vi "test_has_position.vi"() -> ()   [LabVIEW 2022 SP3]
uses:
  <instrlib>/yaq/yaq_labview_error_handler.vi
  <vilib>/Utility/error.llb/Simple Error Handler.vi
panel:
  out "Current Position":dbl
  out "Destination":dbl
  in  "Set Relative":dbl
  in  "Set Position":dbl
  in  "stop":bool
  out "units":string
  out "busy?":bool
  in  "Python path":path=path "C:/ProgramData/Anaconda3/envs/lv4/pythonw.exe"
  in  "Python version":string="3.8.0"
  in  "Python Module Path":path=path "C:/Users/kamey/work/labview/yaq-labview/python/yaqc_labview.py"
  in  "Port":i32=39004
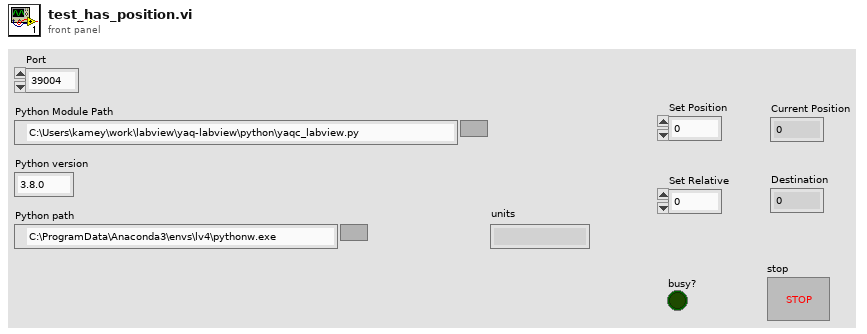
[diagram p1: front panel]
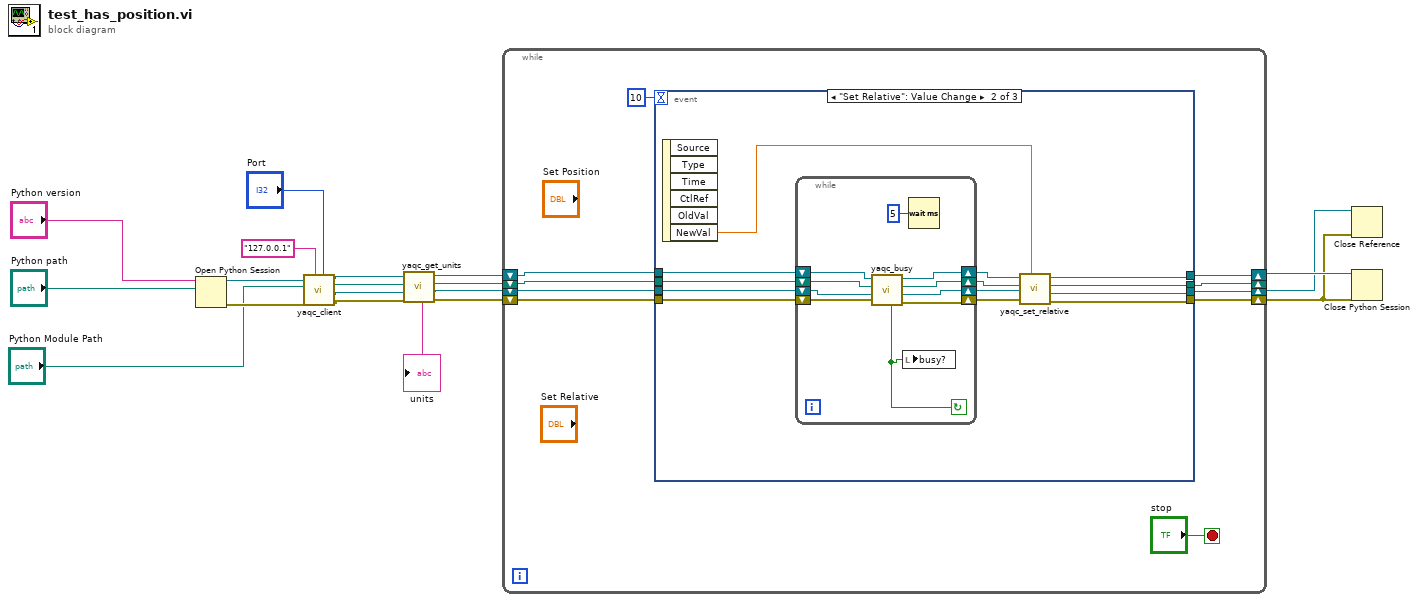
[diagram p0: block diagram]
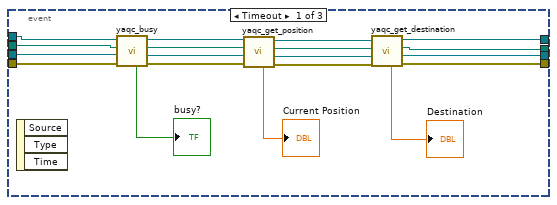
[diagram p2: hidden frame]
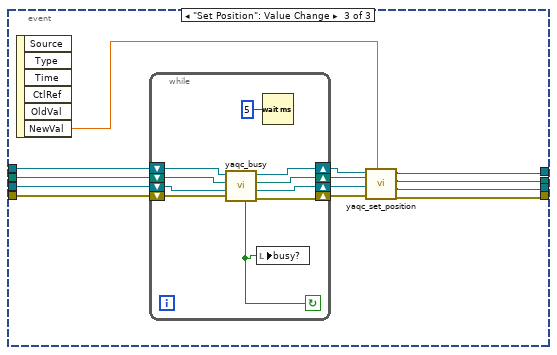
[diagram p3: hidden frame]
diagram:
  n1 = Open Python Session(python version="Python version", python path="Python path") -> (session out=w18:refnum<k35>, error out=w19:errorcluster)  [unwired: 1 in]
  n2 = call "yaqc_client.vi"("Port"="Port", "host ('127.0.0.1')"="127.0.0.1", "error in (no error)"=w19, "Python Module Path"="Python Module Path", "Python Session In"=w18) -> ("error out"=w4:errorcluster, "Yaqc Client"=w3:refnum<k38>, "Python Module Path Out"=w2:path, "Python Session Out"=w1:refnum<k35>)  [unwired: 3 in]
  n3 = call "yaqc_get_units.vi"("error in (no error)"=w4, "Yaqc Client In"=w3, "Python Module Path In"=w2, "Python Session In"=w1) -> ("error out"=w11:errorcluster, "Yaqc Client Out"=w10:refnum<k38>, "Python Module Path Out"=w9:path, "Python Session Out"=w8:refnum<k35>, "units"=→"units":string)  [unwired: 3 in]
  n4 = while {
    shift-right: [w26] -> w6
    shift-left: w11 -> [w28]
    shift-right: [w21] -> w5
    shift-left: w10 -> [w27]
    shift-right: [w22] -> _
    shift-left: w9 -> [w25]
    shift-right: [w23] -> w7
    shift-left: w8 -> [w24]
    stop <- "stop" stop-if-true
    n5 = event shown="[1] \"Set Relative\": Value Change" {
      selector: _ -> [_ _ _]
      dyn-events: _ -> [_ _ _]
      timeout: 10 -> [_ _ _]
      tunnel: w28 -> [w47 w61 w84]
      tunnel: w27 -> [w48 w60 w83]
      tunnel: [w44 w53 w80] -> w26
      tunnel: w25 -> [w43 w59 w82]
      tunnel: w24 -> [w42 w58 w81]
      tunnel: [w35 w50 w73] -> w23
      tunnel: [w34 w51 w75] -> w22
      tunnel: [w33 w52 w77] -> w21
      event Timeout {
        n6 = event-data() -> ()  [unwired: 1 in, 3 out]
        n7 = call "yaqc_busy.vi"("error in (no error)"=w47, "Yaqc Client In"=w48, "Python Module Path In"=w43, "Python Session In"=w42) -> ("error out"=w46:errorcluster, "Yaqc Client Out"=w38:refnum<k38>, "Python Module Path Out"=w39:path, "Python Session Out"=w41:refnum<k35>, "busy?"=→"busy?":bool)  [unwired: 3 in]
        n8 = call "yaqc_get_position.vi"("error in (no error)"=w46, "Yaqc Client In"=w38, "Python Module Path In"=w39, "Python Session In"=w41) -> ("error out"=w45:errorcluster, "Yaqc Client Out"=w37:refnum<k38>, "Python Module Path Out"=w36:path, "Python Session Out"=w40:refnum<k35>, "position"=→"Current Position":dbl)  [unwired: 3 in]
        n9 = call "yaqc_get_destination.vi"("error in (no error)"=w45, "Yaqc Client In"=w37, "Python Module Path In"=w36, "Python Session In"=w40) -> ("error out"=w44:errorcluster, "Yaqc Client Out"=w33:refnum<k38>, "Python Module Path Out"=w34:path, "Python Session Out"=w35:refnum<k35>, "destination"=→"Destination":dbl)  [unwired: 3 in]
      }
      event "Set Relative": Value Change {
        n10 = event-data() -> ("NewVal"=w49:dbl)  [unwired: 1 in, 5 out]
        n11 = while {
          shift-right: [w64] -> w57
          shift-left: w61 -> [w71]
          shift-right: [w65] -> w56
          shift-left: w60 -> [w70]
          shift-right: [w66] -> w55
          shift-left: w59 -> [w69]
          shift-right: [w67] -> w54
          shift-left: w58 -> [w68]
          stop <- w62 continue-if-true
          n12 = call "yaqc_busy.vi"("error in (no error)"=w71, "Yaqc Client In"=w70, "Python Module Path In"=w69, "Python Session In"=w68) -> ("error out"=w64:errorcluster, "Yaqc Client Out"=w65:refnum<k38>, "Python Module Path Out"=w66:path, "Python Session Out"=w67:refnum<k35>, "busy?"=w62:bool)  [unwired: 3 in]
          n13 = local write "busy?"(w62) -> ()
          n14 = Wait (ms)(milliseconds to wait=u32 5) -> ()  [unwired: 1 out]
        }
        n15 = call "yaqc_set_relative.vi"("rel. position"=w49, "error in (no error)"=w57, "Yaqc Client In"=w56, "Python Module Path In"=w55, "Python Session In"=w54) -> ("error out"=w53:errorcluster, "Yaqc Client Out"=w52:refnum<k38>, "Python Module Path Out"=w51:path, "Python Session Out"=w50:refnum<k35>)  [unwired: 3 in]
      }
      event "Set Position": Value Change {
        n16 = event-data() -> ("NewVal"=w72:dbl)  [unwired: 1 in, 5 out]
        n17 = while {
          shift-right: [w87] -> w79
          shift-left: w84 -> [w94]
          shift-right: [w88] -> w78
          shift-left: w83 -> [w93]
          shift-right: [w89] -> w76
          shift-left: w82 -> [w92]
          shift-right: [w90] -> w74
          shift-left: w81 -> [w91]
          stop <- w85 continue-if-true
          n18 = call "yaqc_busy.vi"("error in (no error)"=w94, "Yaqc Client In"=w93, "Python Module Path In"=w92, "Python Session In"=w91) -> ("error out"=w87:errorcluster, "Yaqc Client Out"=w88:refnum<k38>, "Python Module Path Out"=w89:path, "Python Session Out"=w90:refnum<k35>, "busy?"=w85:bool)  [unwired: 3 in]
          n19 = local write "busy?"(w85) -> ()
          n20 = Wait (ms)(milliseconds to wait=u32 5) -> ()  [unwired: 1 out]
        }
        n21 = call "yaqc_set_position.vi"("position"=w72, "error in (no error)"=w79, "Yaqc Client In"=w78, "Python Module Path In"=w76, "Python Session In"=w74) -> ("error out"=w80:errorcluster, "Yaqc Client Out"=w77:refnum<k38>, "Python Module Path Out"=w75:path, "Python Session Out"=w73:refnum<k35>)  [unwired: 3 in]
      }
    }
  }
  n22 = Close Reference(reference=w5, error in (no error)=w6) -> ()  [unwired: 1 out]
  n23 = Close Python Session(session in=w7, error in=w6) -> ()  [unwired: 1 out]
